vi "Setup SmartMotor.vi"(0 "reference in":refnum<class "SmartMotor.lvclass">, 1 "SmartMotor Chain VISA Session":refnum<visa-resource-name>, 3 "SmartMotor Chain Address":i16 max=10 step=1, 4 "Screwdriver Torque Limit":i32=1500 format="%#.0f", 5 "error in (no error)":errorcluster) -> (14 "reference out":refnum<class "SmartMotor.lvclass">, 15 "SmartMotor Chain VISA Session OUT":refnum<visa-resource-name>, 19 "error out":errorcluster)   [LabVIEW 2017, in "SmartMotor.lvclass"]
uses:
  SmartMotor.lvclass
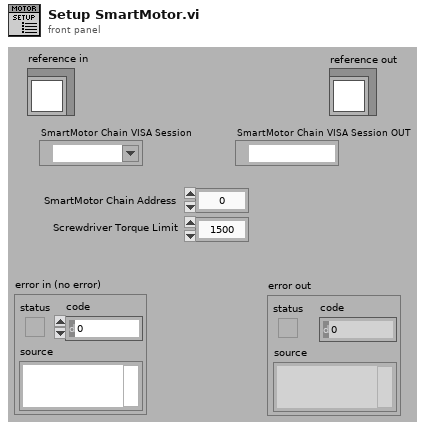
[diagram p1: front panel]
types:
  T1 = typedef "SmartMotor.lvclass/ObjectAttributes.ctl" = cluster{"SmartMotor Chain VISA Resource":refnum<visa-resource-name>, "SmartMotor Chain Address":i16, "Motor Absolute Position":i32, "Motor Relative Position":i32, "Motor Torque":i32, "Motor Voltage":i32, "Screwdriver Engaged":bool, "Screwdriver Torque Limit":i32, "Torque Monitor On/Off Status":bool, "Torque Monitor VI Reference":refnum<vi>, "Absolute Motor Torque (Filtered)":dbl, "SmartMotor Status":T2, "SmartMotor Error":T3}
  T2 = typedef "SmartMotor.lvclass/SmartMotor Status.ctl" = enum8{"Stopped", "Moving"}
  T3 = typedef "SmartMotor.lvclass/SmartMotor Error.ctl" = enum8{"None", "Read Error", "Low Voltage"}
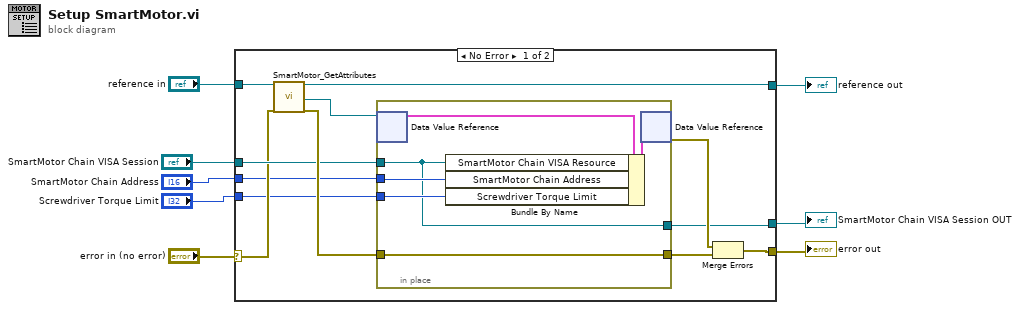
[diagram p0: block diagram]
diagram:
  n1 = case shown="No Error" "error in (no error)" {
    selector: "error in (no error)" -> [w12 w28]
    tunnel: [w17 w28] -> w7
    tunnel: [w18 w27] -> w5
    tunnel: "reference in" -> [w20 w27]
    tunnel: "SmartMotor Chain VISA Session" -> [w13 _]
    tunnel: "SmartMotor Chain Address" -> [w11 _]
    tunnel: "Screwdriver Torque Limit" -> [w10 _]
    tunnel: [w9 _] -> w1
    frame No Error {
      n2 = call "SmartMotor_GetAttributes.vi"("reference in"=w20, "error in (no error)"=w12) -> ("reference out"=w18:refnum<class "SmartMotor.lvclass">, "DataRef"=w16:refnum<data-value>, "error out"=w15:errorcluster)  [unwired: 14 in, 1 out]
      n3 = in-place {
        in-place-border: w15 -> [w24]
        in-place-border: [w24] -> w14
        in-place-border: w13 -> [w21]
        in-place-border: w11 -> [w23]
        in-place-border: w10 -> [w22]
        in-place-border: [w21] -> w9
        n4 = in-place-dvr #1(w16) -> (w25:T1)  [unwired: 1 out]
        n5 = Bundle By Name(cluster=w25, "SmartMotor Chain VISA Resource"=w21, "SmartMotor Chain Address"=w23, "Screwdriver Torque Limit"=w22) -> (w26:T1)
        n6 = in-place-dvr #1(w26) -> (w19:errorcluster)  [unwired: 1 out]
      }
      n7 = Merge Errors(w19, w14) -> (w17:errorcluster)
    }
    frame Error {
    }
  }
  "error out" <- w7
  "reference out" <- w5
  "SmartMotor Chain VISA Session OUT" <- w1
